vi "Write Tab Control.vi"(8 "error in (no error)":errorcluster, 10 "Tab Control":refnum<vi>, 11 "Function UI in":refnum<class "Controller UI.lvclass">) -> (0 "error out":errorcluster, 3 "Function UI out":refnum<class "Controller UI.lvclass">)   [LabVIEW 2016, in "Controller UI.lvlib" / "Controller UI.lvclass"]
uses:
  <userlib>/Common Components/Controller UI/Controller UI.lvclass
  <userlib>/Common Components/Controller UI/Controller UI.lvclass/Controller UI.ctl
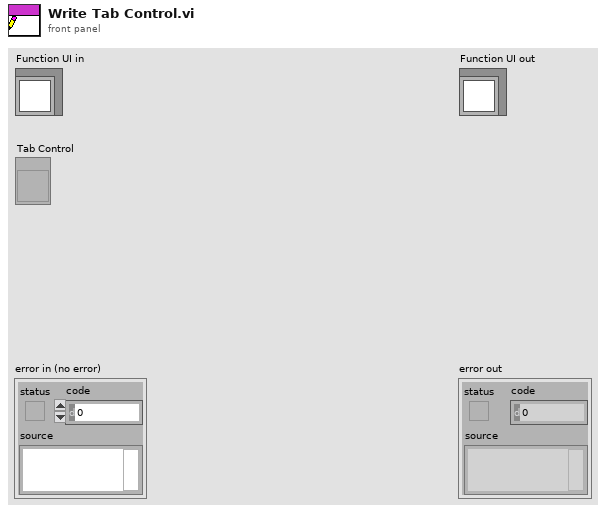
[diagram p1: front panel]
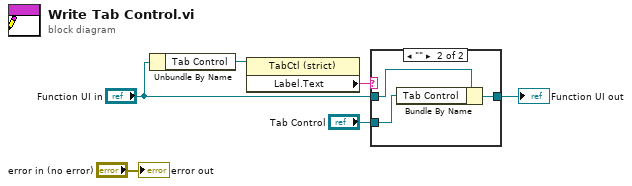
[diagram p0: block diagram]
diagram:
  n1 = Unbundle By Name("Function UI in") -> ("Tab Control"=w3:refnum<vi>)
  n2 = property class="TabCtl (strict)"(reference=w3) -> ("Label.Text"=w1:string)  [unwired: 1 in, 2 out]
  n3 = case shown="\"\"" w1 {
    tunnel: [w7 w9] -> w6
    tunnel: "Function UI in" -> [w7 w10]
    tunnel: "Tab Control" -> [_ w8]
    frame Default {
    }
    frame "" {
      n4 = Bundle By Name(cluster=w10, "Tab Control"=w8) -> (w9:refnum<class "Controller UI.lvclass">)
    }
  }
  "Function UI out" <- w6
  "error out" <- "error in (no error)"
